vi "SMO.Example.GetDependencies.vi"(8 "error in (no error)":errorcluster, 11 "SMO.Example":refnum<class "SMO.TopLevel.lvclass">) -> (0 "error out":errorcluster, 2 "Dependencies":T1, 3 "SMO.Example out":refnum<class "SMO.TopLevel.lvclass">)   [LabVIEW 2013, in "SMO.TopLevel.lvclass"]
doc: "---------------------------------------------------------------\nJKI State Machine Objects™\nhttp://jki.net/state-machine-objects/\nCopyright (C) 2005-2015, JKI <info@jki.net>\nALL RIGHTS RESERVED"
uses:
  SMO.TopLevel.lvclass
  Typedefs/Dependencies--Cluster.ctl
  SMO.A/SMO.A.lvclass
  src/SMO/SMO.lvclass
panel:
  # "For instructions on how to use the JKI State Machine Objects, examples and video tutorials, visit:\nhttp://jki.net/state-machine-objects/\n\nJKI State Machine Objects™\nhttp://jki.net/state-machine-objects/\nCopyright (C) 2005-2015, JKI <info@jki.net>\nALL RIGHTS RESERVED"
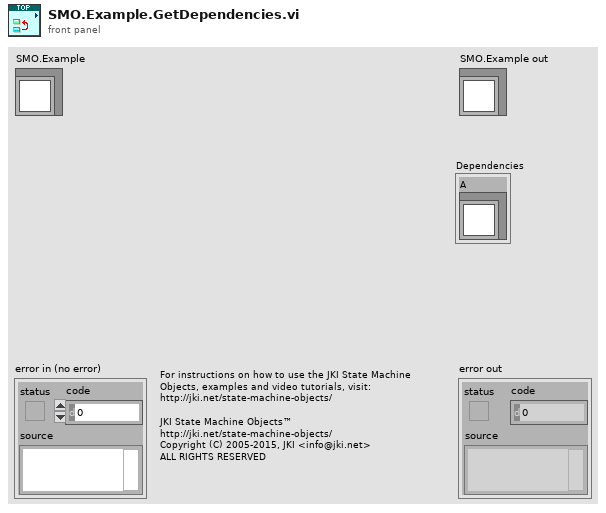
[diagram p1: front panel]
types:
  T1 = typedef "SMO.TopLevel.lvclass/Dependencies--Cluster.ctl" = cluster{"A":refnum<class "SMO.A.lvclass">}
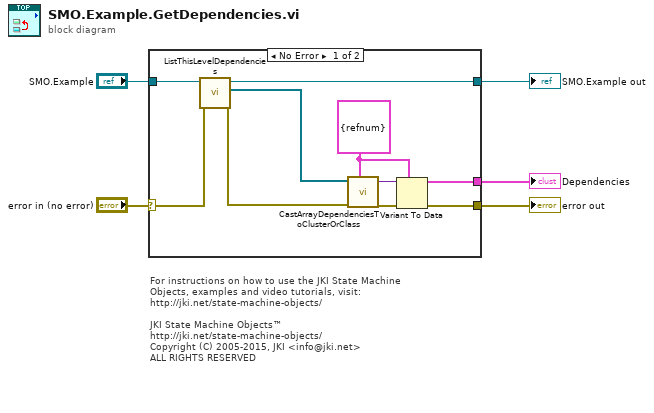
[diagram p0: block diagram]
diagram:
  # "For instructions on how to use the JKI State Machine Objects, examples and video tutorials, visit:\nhttp://jki.net/state-machine-objects/\n\nJKI State Machine Objects™\nhttp://jki.net/state-machine-objects/\nCopyright (C) 2005-2015, JKI <info@jki.net>\nALL RIGHTS RESERVED"
  n1 = case shown="No Error" "error in (no error)" {
    selector: "error in (no error)" -> [w7 w16]
    tunnel: "SMO.Example" -> [w15 w17]
    tunnel: [w6 w16] -> w4
    tunnel: [w14 w17] -> w3
    tunnel: [w9 _] -> w1
    frame No Error {
      w10 = T1 {"A"=refnum} ("Dependencies")
      n2 = call "ListThisLevelDependencies.vi"("error in (no error)"=w7, "SMO in"=w15) -> ("error out"=w8:errorcluster, "[My Dependencies]"=w13:refnum<class "SMO.lvclass">[], "SMO out"=w14:refnum<class "SMO.TopLevel.lvclass">)  [unwired: 7 in]
      n3 = call "CastArrayDependenciesToClusterOrClass.vi"("Dependency Type (Class|Cluster)"=w10, "error in (no error)"=w8, "[Dependencies]"=w13) -> ("error out"=w12:errorcluster, "Dependencies output"=w11:variant)  [unwired: 7 in]
      n4 = Variant To Data(error in=w12, type=w10, Variant=w11) -> (data=w9:T1, error out=w6:errorcluster)
    }
    frame Error {
    }
  }
  "error out" <- w4
  "SMO.Example out" <- w3
  "Dependencies" <- w1
